vi "Tidal Eng-String Data.vi"(8 "error in (no error)":errorcluster, 11 "Tenney Environmental Chamber Data Input":T1) -> (0 "error out":errorcluster, 2 "Tenney Data":string[][](array[string]), 3 "Tenney Environmental Chamber Data Output":T1)   [LabVIEW 2023]
uses:
  Type Definitions/Tenney Environmental Chamber Data.ctl
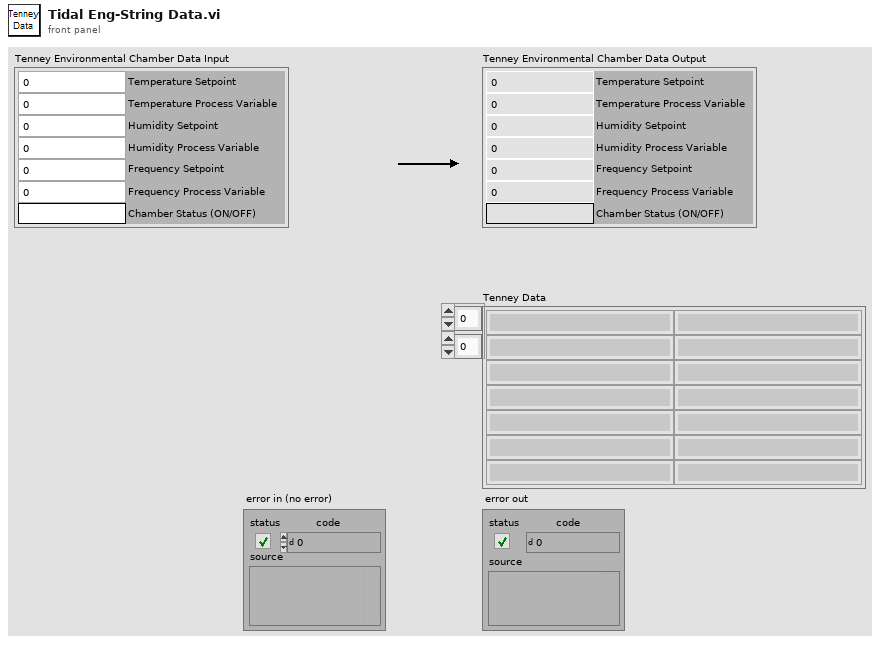
[diagram p1: front panel]
types:
  T1 = typedef "Tenney Environmental Chamber Data.ctl" = cluster{"Temperature Setpoint":dbl, "Temperature Process Variable":dbl, "Humidity Setpoint":dbl, "Humidity Process Variable":dbl, "Frequency Setpoint":dbl, "Frequency Process Variable":dbl, "Chamber Status (ON/OFF)":string}
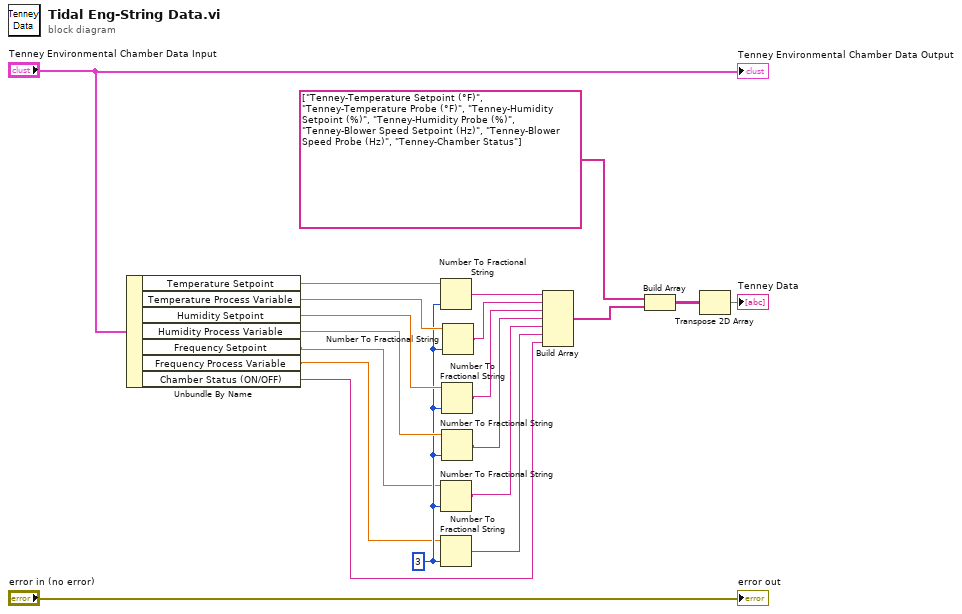
[diagram p0: block diagram]
diagram:
  w7 = i16 3 ("precision (6)")
  n1 = Unbundle By Name("Tenney Environmental Chamber Data Input") -> ("Temperature Setpoint"=w19:dbl, "Temperature Process Variable"=w18:dbl, "Humidity Setpoint"=w17:dbl, "Humidity Process Variable"=w16:dbl, "Frequency Setpoint"=w6:dbl, "Frequency Process Variable"=w5:dbl, "Chamber Status (ON/OFF)"=w2:string)
  n2 = Number To Fractional String(number=w19, precision (6)=w7) -> (F-format string=w15:string)  [unwired: 2 in]
  n3 = Number To Fractional String(number=w6, precision (6)=w7) -> (F-format string=w4:string)  [unwired: 2 in]
  n4 = Number To Fractional String(number=w5, precision (6)=w7) -> (F-format string=w3:string)  [unwired: 2 in]
  n5 = Number To Fractional String(number=w17, precision (6)=w7) -> (F-format string=w13:string)  [unwired: 2 in]
  n6 = Number To Fractional String(number=w16, precision (6)=w7) -> (F-format string=w12:string)  [unwired: 2 in]
  n7 = Number To Fractional String(number=w18, precision (6)=w7) -> (F-format string=w14:string)  [unwired: 2 in]
  n8 = Build Array(w15, w14, w13, w12, w4, w3, w2) -> (w10:string[])
  n9 = Build Array(string[] ["Tenney-Temperature Setpoint (°F)", "Tenney-Temperature Probe (°F)", "Tenney-Humidity Setpoint (%)", "Tenney-Humidity Probe (%)", "Tenney-Blower Speed Setpoint (Hz)", "Tenney-Blower Speed Probe (Hz)", "Tenney-Chamber Status"], w10) -> (w9:string[][])
  n10 = Transpose 2D Array(2D array=w9) -> (transposed array=→"Tenney Data":string[][])
  "Tenney Environmental Chamber Data Output" <- "Tenney Environmental Chamber Data Input"
  "error out" <- "error in (no error)"
